vi "test_Configure Response_Variable Duplicate Error.vi"(8 "error in (no error)":errorcluster, 11 "TestCase in":refnum<class "Instrument Addon Scripting API Messages Unit Tests.lvclass">) -> (0 "error out":errorcluster, 3 "TestCase out":refnum<class "Instrument Addon Scripting API Messages Unit Tests.lvclass">)   [LabVIEW 2018, in "Instrument Addon Scripting API Messages Unit Tests.lvclass"]
uses:
  Instrument Addon Scripting API Messages Unit Tests.lvclass
  APIs/Scripting API/TypeDefs/Wait Response Settings.ctl
  APIs/Scripting API/TypeDefs/Linked Channel.ctl
  <vilib>/NI Veristand/Custom Device API/Custom Device Item Ref.ctl
  Instrument Addon Scripting API Messages Unit Tests.lvclass/Instrument Addon Scripting API Messages Unit Tests.ctl
  Addon/Addon Shared/SubVIs/Constants.vi
  <vilib>/NI/NI VeriStand Advanced SysDef API/_SubVIs/SysDef.Search.GUID.vi
  APIs/Scripting API/Messages/Configure Response - Wait (sec).vi
  <vilib>/addons/_JKI Toolkits/VI Tester/TestCase.llb/TestCase.lvclass
  Instrument Addon Scripting API Test Assets/Instrument Addon Scripting API Test Assets.lvclass
  APIs/Scripting API/Instrument Addon Scripting API.lvlib
  <vilib>/NI Veristand/Custom Device API/Custom Device API.lvlib
  <vilib>/NI/NI VeriStand Advanced SysDef API/SysDef API/Advanced System Definition.lvlib
  Addon/Addon Shared/Instrument Addon Shared.lvlib
  C:/Program Files (x86)/National Instruments/LabVIEW 2018/vi.lib/addons/_JKI Toolkits/VI Tester/TestCase.llb/TestCase.lvclass
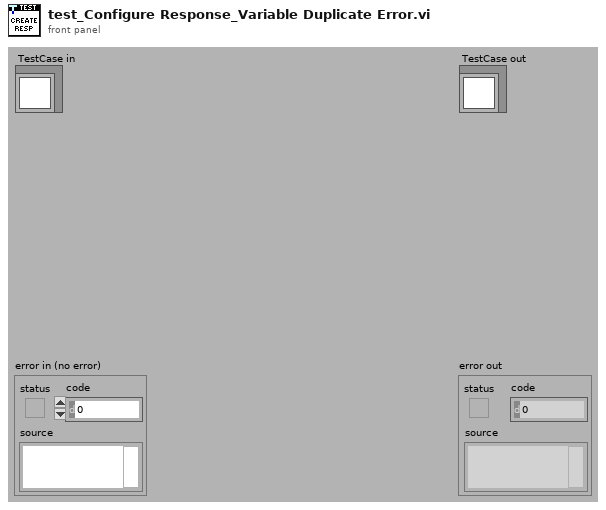
[diagram p1: front panel]
types:
  T1 = typedef "Instrument Addon Scripting API.lvlib/Wait Response Settings.ctl" = cluster{"Response Format":string, "Linked Channels":T2[], "Wait value (sec)":dbl, "Use Wait Channel":bool, "Channel Refnum":T3}
  T2 = typedef "Instrument Addon Scripting API.lvlib/Linked Channel.ctl" = cluster{"Variable Name":string, "Channel Refnum":T3}
  T3 = typedef "Custom Device API.lvlib/Custom Device Item Ref.ctl" = u64
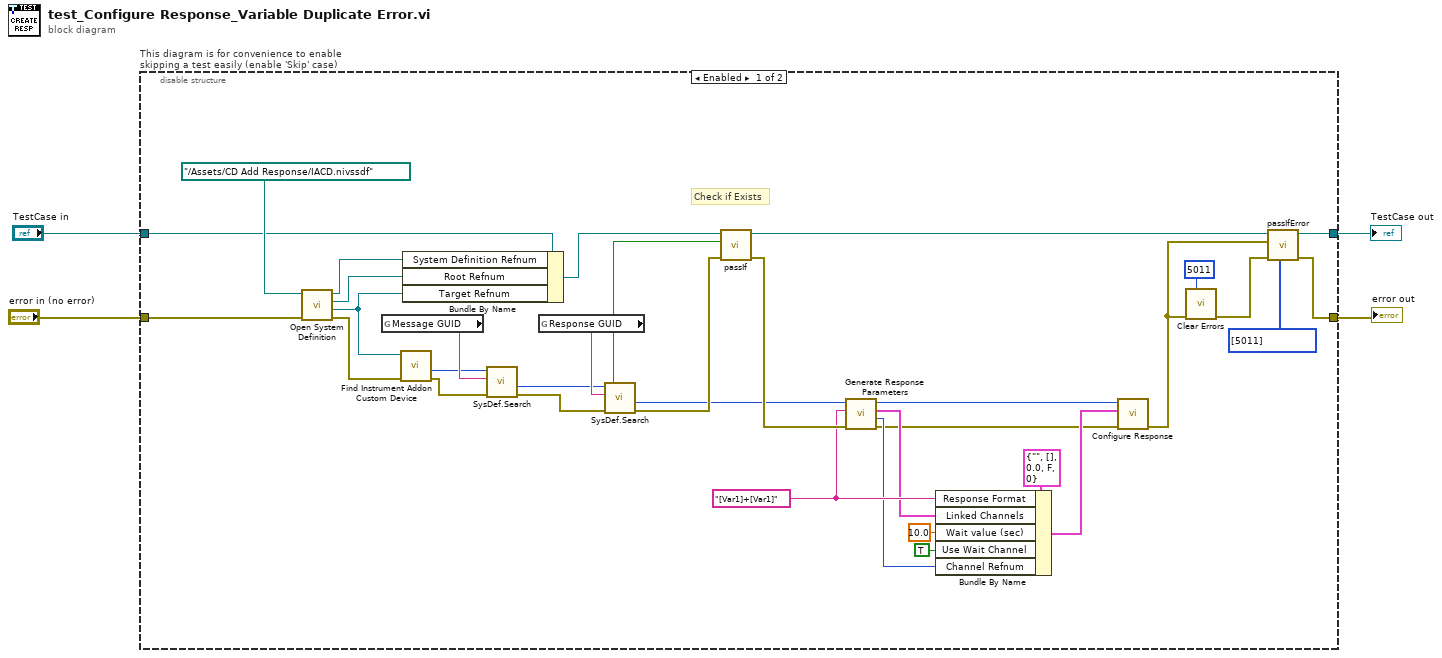
[diagram p0: block diagram]
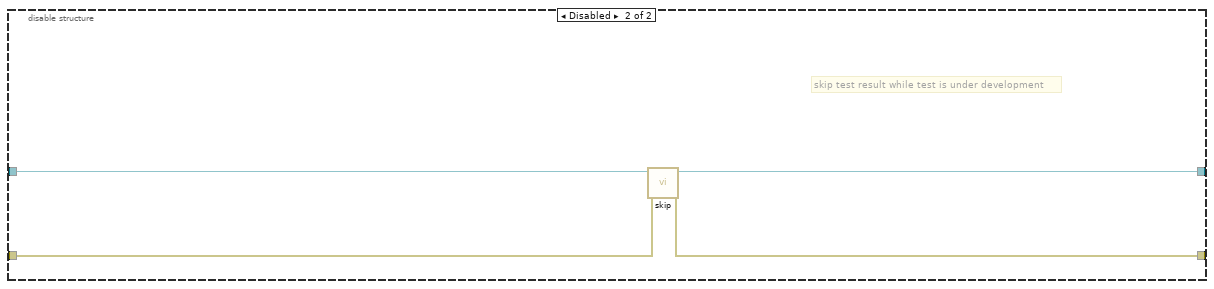
[diagram p2: hidden frame]
diagram:
  n1 = disable-structure "This diagram is for convenience to enable skipping a test easily (enable 'Skip' case)" shown="Enabled" {
    disable-tunnel: "TestCase in" -> [w12 w42]
    disable-tunnel: [w29 w40] -> w1
    disable-tunnel: [w28 w41] -> w3
    disable-tunnel: "error in (no error)" -> [w37 w39]
    frame Enabled {
      w19 = "[Var1]+[Var1]" ("Response Format")
      # "Check if Exists"
      n2 = call "Open System Definition.vi"("error in (no error)"=w37, "System Definition File"=path "../Assets/CD Add Response/IACD.nivssdf" ("SDF file")) -> ("error out"=w36:errorcluster, "Target Refnum"=w10:refnum<k24>, "Root Refnum"=w9:refnum<k24>, "System Definition Refnum"=w8:refnum<k24>)  [unwired: 6 in]
      n3 = global read "Constants.vi" "Message GUID"() -> (w24:string)
      n4 = call "Find Instrument Addon Custom Device.vi"("error in"=w36, "target in"=w10) -> ("error out"=w25:errorcluster, "NodeID"=w21:u64)  [unwired: 7 in, 1 out]
      n5 = Bundle By Name(cluster=w12, "System Definition Refnum"=w8, "Root Refnum"=w9, "Target Refnum"=w10) -> (w11:refnum<class "Instrument Addon Scripting API Messages Unit Tests.lvclass">)
      n6 = call-poly <vilib>:"SysDef.Search.vi"("error in (no error)"=w25, "GUID"=w24, "nodeID"=w21) -> ("error out"=w22:errorcluster, "Value out"=w23:u64)  [unwired: 5 in, 2 out]
      n7 = global read "Constants.vi" "Response GUID"() -> (w34:string)
      n8 = call-poly <vilib>:"SysDef.Search.vi"("error in (no error)"=w22, "GUID"=w34, "nodeID"=w23) -> ("error out"=w14:errorcluster, "Value out"=w13:u64, "Found?"=w33:bool)  [unwired: 5 in, 1 out]
      n9 = call-dynamic "passIf.vi"("error in (no error)"=w14, "pass"=w33, "TestCase in"=w11) -> ("error out"=w20:errorcluster, "TestCase out"=w30:refnum<class "Instrument Addon Scripting API Messages Unit Tests.lvclass">)  [unwired: 7 in]
      n10 = call "Generate Response Parameters.vi"("Error In"=w20, "Response String"=w19, "Response Channel in"=w13) -> ("Error Out"=w15:errorcluster, "Wait Channel Ref out"=w17:T3, "Linked Channels"=w18:T2[], "Response Channel out"=w5:T3)  [unwired: 5 in]
      n11 = Bundle By Name(cluster=T1 {"Response Format"="", "Linked Channels"=[], "Wait value (sec)"=0.0, "Use Wait Channel"=FALSE, "Channel Refnum"=0} ("Settings"), "Response Format"=w19, "Linked Channels"=w18, "Wait value (sec)"=10.0, "Use Wait Channel"=TRUE ("Use Byte Count channel"), "Channel Refnum"=w17) -> (w16:T1)
      n12 = call-poly "Configure Response.vi"("error in (no error)"=w15, "settings"=w16, "reponse refnum in"=w5) -> ("error out"=w7:errorcluster)  [unwired: 7 in, 1 out]
      n13 = call <vilib>:"Clear Errors.vi"("error in (no error)"=w7, "specific error code to clear (0: all)"=5011) -> ("error out"=w26:errorcluster)  [unwired: 4 in, 1 out]
      n14 = call-dynamic "passIfError.vi"("passing error codes (default = any error code)"=i32[] [5011], "error in (no error)"=w26, "error"=w7, "TestCase in"=w30) -> ("error out"=w28:errorcluster, "TestCase out"=w29:refnum<class "Instrument Addon Scripting API Messages Unit Tests.lvclass">)  [unwired: 6 in]
    }
    frame Disabled {
      # "skip test result while test is under development"
      n15 = call <vilib>:"skip.vi"("error in (no error)"=w39, "TestCase in"=w42) -> ("error out"=w41:errorcluster, "TestCase out"=w40:refnum<class "Instrument Addon Scripting API Messages Unit Tests.lvclass">)  [unwired: 8 in]
    }
  }
  "error out" <- w3
  "TestCase out" <- w1
